vi "probe_pol_mod.vi"() -> ()   [LabVIEW 2011]
uses:
  <vilib>/express/express arith-compare/Formula/XNode/ExpressFormulaBlockNode.xnode
panel:
  out "Right AC":dbl format="%#_5g"
  out "Left AC":dbl format="%#_5g"
  in  "Extract Tone?":bool
  out "Right Amplitude":dbl
  out "Right Freq":dbl
  out "Left Amplitude":dbl
  out "Left Freq":dbl
  out "Pump Status":bool
  in  "Pump Power On?":bool
  out "Right Peak to Peak":dbl
  out "Left Peak to Peak":dbl
  out "Right Ratio":dbl
  out "Left Ratio":dbl
  in  "Shutter":bool
  out "r":dbl
  in  "Number Right Samples":i32=1100
  out "Right Zero Pump On":dbl
  out "Left Zero Pump On":dbl
  out "Waveform Chart":dbl(graph)
  out "Polarization":dbl
  in  "Set Zero":bool
  out "Right Zero":dbl
  out "Left Zero":dbl
  in  "Number Left Samples":i32=2000
  out "Right Mean":dbl format="%#_5g"
  out "Left Mean":dbl format="%#_5g"
  out "Signals":dynamicdata(graph) caption="Section"
  in  "High Signal Start":i32=100 caption="Begin Sample"
  in  "Low Signal Start":i32=1000 caption="Begin Sample"
  in  "stop":bool
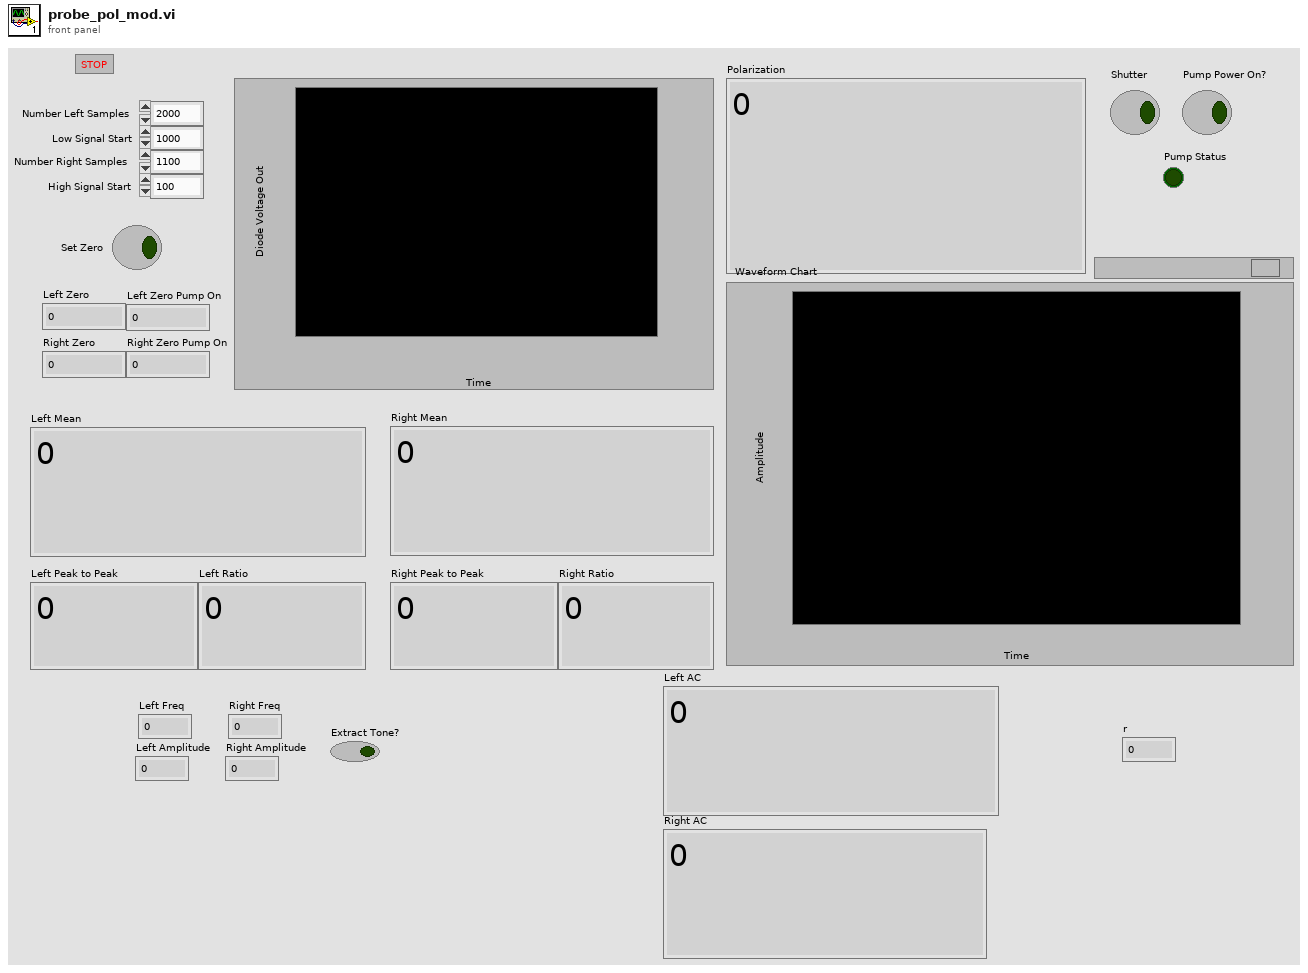
[diagram p1: front panel]
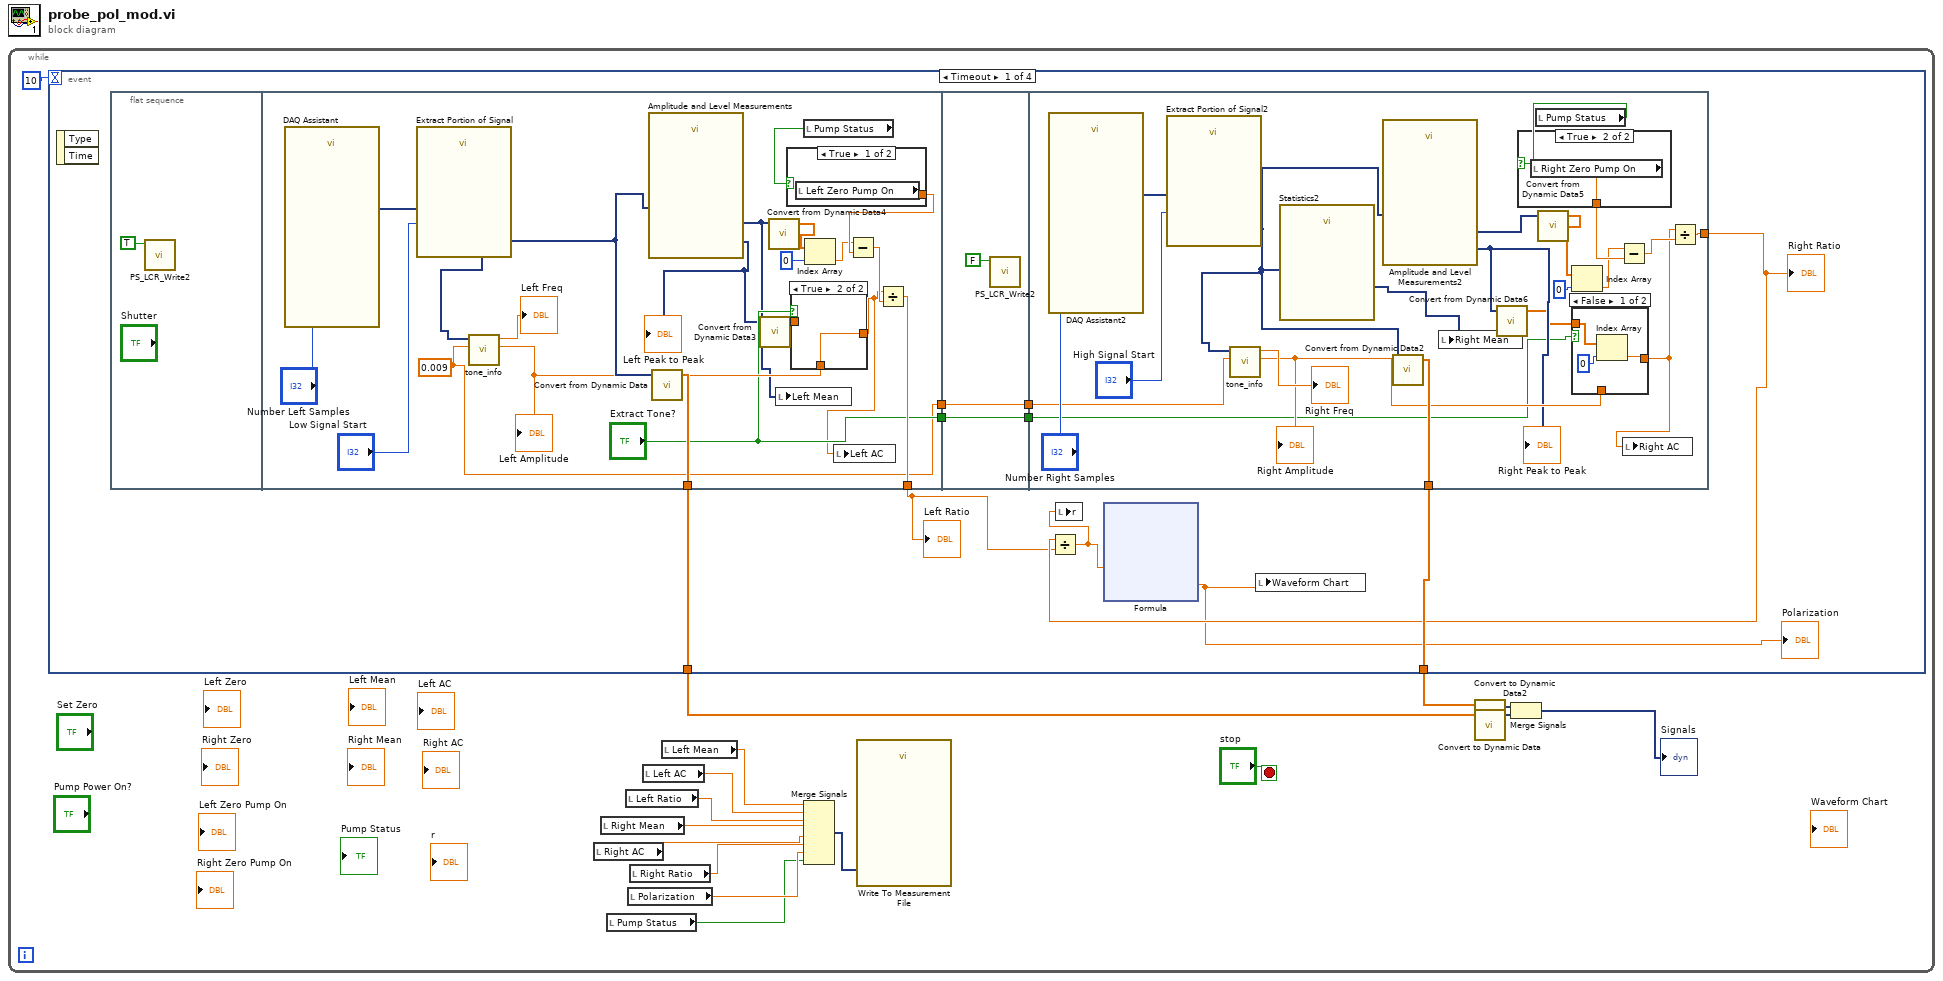
[diagram p0: block diagram]
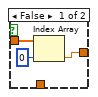
[diagram p2: hidden frame]
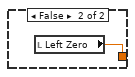
[diagram p3: hidden frame]
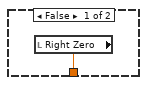
[diagram p5: hidden frame]
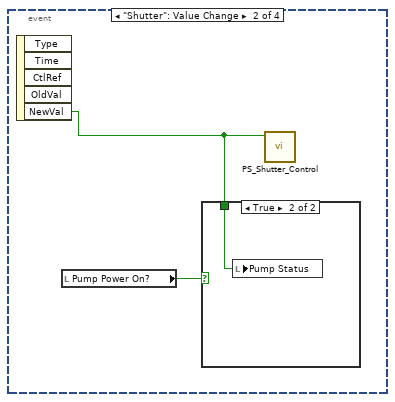
[diagram p6: hidden frame]
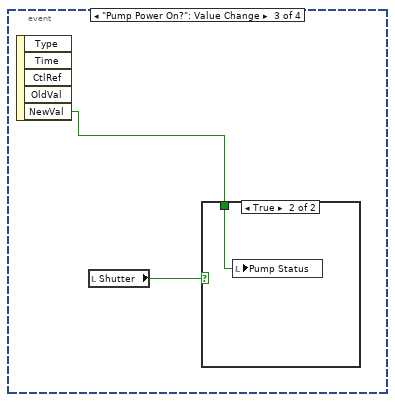
[diagram p8: hidden frame]
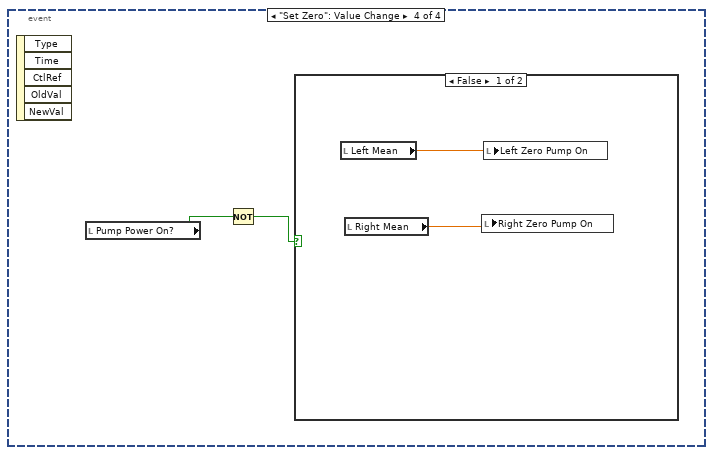
[diagram p10: hidden frame]
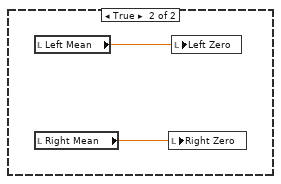
[diagram p11: hidden frame]
diagram:
  n1 = while {
    stop <- "stop" stop-if-true
    n2 = event shown="[0] Timeout" {
      selector: _ -> [_ _ _ _]
      dyn-events: _ -> [_ _ _ _]
      timeout: 10 -> [_ _ _ _]
      tunnel: [w26 _ _ _] -> w14
      tunnel: [w25 _ _ _] -> w12
      event Timeout {
        n3 = event-data() -> ()  [unwired: 1 in, 2 out]
        n4 = flat-sequence {
          tunnel: [w52] -> w26
          tunnel: [w51] -> w21
          tunnel: ["Extract Tone?"] -> w22
          tunnel: [w36] -> w17
          tunnel: [w63] -> w23
          tunnel: w22 -> [w63]
          tunnel: [w62] -> w18
          tunnel: w17 -> [w62]
          tunnel: [w83] -> w25
          tunnel: [w80] -> w24
          tunnel: w23 -> [w67]
          tunnel: w18 -> [w65]
          frame #0 {
            n5 = call "PS_LCR_Write2.vi"("On/Off"=TRUE) -> ()  [unwired: 10 in, 1 out]
          }
          frame #1 {
            w36 = 0.009 ("threshold")
            n6 = call "DAQ Assistant"("number of samples"="Number Left Samples") -> ("data"=w54:dynamicdata)  [unwired: 16 in, 2 out]
            n7 = call "Extract Portion of Signal"("Begin Sample"="Low Signal Start", "Signals"=w54) -> ("Section"=w47:dynamicdata)  [unwired: 8 in, 1 out]
            n8 = call "tone_info.vi"("threshold"=w36, "time signal in"=w47) -> ("amplitude"=w45:dbl, "frequency"=→"Left Freq":dbl)  [unwired: 7 in, 1 out]
            "Left Amplitude" <- w45
            n9 = call "Amplitude and Level Measurements"("Signals"=w47) -> ("Mean (DC)"=w41:dynamicdata, "Peak to Peak"=w42:dynamicdata)  [unwired: 12 in, 1 out]
            "Left Peak to Peak" <- w42
            n10 = call "Convert from Dynamic Data"("Dynamic Data Type"=w47) -> ("Array"=w52:dbl[])  [unwired: 3 in]
            n11 = call "Convert from Dynamic Data3"("Dynamic Data Type"=w42) -> ("Array"=w43:dbl[])  [unwired: 3 in]
            n12 = call "Convert from Dynamic Data4"("Dynamic Data Type"=w41) -> ("Array"=w39:dbl[])  [unwired: 3 in]
            n13 = local write "Left Mean"(w41) -> ()
            n14 = case shown="True" "Extract Tone?" {
              tunnel: [w57 w59] -> w37
              tunnel: w45 -> [_ w59]
              tunnel: w43 -> [w58 _]
              frame False {
                n15 = Index Array(array=w58, index=0) -> (element=w57:dbl)
              }
              frame True {
              }
            }
            n16 = local read "Pump Status"() -> (w50:bool)
            n17 = case shown="True" w50 {
              tunnel: [w60 w61] -> w49
              frame True {
                n18 = local read "Left Zero Pump On"() -> (w60:dbl)
              }
              frame False {
                n19 = local read "Left Zero"() -> (w61:dbl)
              }
            }
            n20 = Index Array(array=w39, index=0) -> (element=w40:dbl)
            n21 = local write "Left AC"(w37) -> ()
            n22 = Subtract(x=w40, y=w49) -> (x-y=w48:dbl)
            n23 = Divide(x=w37, y=w48) -> (x/y=w51:dbl)
          }
          frame #2 {
            n24 = call "PS_LCR_Write2.vi"("On/Off"=FALSE) -> ()  [unwired: 10 in, 1 out]
          }
          frame #3 {
            n25 = call "DAQ Assistant2"("number of samples"="Number Right Samples") -> ("data"=w84:dynamicdata)  [unwired: 16 in, 2 out]
            n26 = call "Extract Portion of Signal2"("Begin Sample"="High Signal Start", "Signals"=w84) -> ("Section"=w75:dynamicdata)  [unwired: 8 in, 1 out]
            n27 = call "tone_info.vi"("threshold"=w65, "time signal in"=w75) -> ("amplitude"=w70:dbl, "frequency"=→"Right Freq":dbl)  [unwired: 7 in, 1 out]
            "Right Amplitude" <- w70
            n28 = call "Statistics2"("Signals"=w75) -> ("Arithmetic Mean"=w82:dynamicdata)  [unwired: 24 in, 2 out]
            n29 = call "Amplitude and Level Measurements2"("Signals"=w75) -> ("Mean (DC)"=w72:dynamicdata, "Peak to Peak"=w69:dynamicdata)  [unwired: 12 in, 1 out]
            "Right Peak to Peak" <- w69
            n30 = call "Convert from Dynamic Data2"("Dynamic Data Type"=w75) -> ("Array"=w83:dbl[])  [unwired: 3 in]
            n31 = local write "Right Mean"(w82) -> ()
            n32 = call "Convert from Dynamic Data6"("Dynamic Data Type"=w69) -> ("Array"=w68:dbl[])  [unwired: 3 in]
            n33 = local read "Pump Status"() -> (w79:bool)
            n34 = case shown="True" w79 {
              tunnel: [w90 w91] -> w77
              frame False {
                n35 = local read "Right Zero"() -> (w90:dbl)
              }
              frame True {
                n36 = local read "Right Zero Pump On"() -> (w91:dbl)
              }
            }
            n37 = call "Convert from Dynamic Data5"("Dynamic Data Type"=w72) -> ("Array"=w74:dbl[])  [unwired: 3 in]
            n38 = Index Array(array=w74, index=0) -> (element=w71:dbl)
            n39 = case shown="False" w67 {
              tunnel: [w87 w89] -> w66
              tunnel: w70 -> [_ w89]
              tunnel: w68 -> [w86 _]
              frame False {
                n40 = Index Array(array=w86, index=0) -> (element=w87:dbl)
              }
              frame True {
              }
            }
            n41 = Subtract(x=w71, y=w77) -> (x-y=w78:dbl)
            n42 = local write "Right AC"(w66) -> ()
            n43 = Divide(x=w66, y=w78) -> (x/y=w80:dbl)
          }
        }
        n44 = Divide(x=w24, y=w21) -> (x/y=w20:dbl)
        n45 = local write "r"(w20) -> ()
        n46 = xnode "Formula"("r"=w20) -> ("Result"=w19:dbl)  [unwired: 1 in, 1 out]
        "Polarization" <- w19
        n47 = local write "Waveform Chart"(w19) -> ()
        "Left Ratio" <- w21
        "Right Ratio" <- w24
      }
      event "Shutter": Value Change {
        n48 = event-data() -> ("NewVal"=w93:bool)  [unwired: 1 in, 4 out]
        n49 = local read "Pump Power On?"() -> (w92:bool)
        n50 = case shown="True" w92 {
          tunnel: w93 -> [_ w94]
          frame False {
          }
          frame True {
            n51 = local write "Pump Status"(w94) -> ()
          }
        }
        n52 = call "PS_Shutter_Control.vi"("On/Off"=w93) -> ()  [unwired: 10 in, 1 out]
      }
      event "Pump Power On?": Value Change {
        n53 = event-data() -> ("NewVal"=w96:bool)  [unwired: 1 in, 4 out]
        n54 = local read "Shutter"() -> (w95:bool)
        n55 = case shown="True" w95 {
          tunnel: w96 -> [_ w97]
          frame False {
          }
          frame True {
            n56 = local write "Pump Status"(w97) -> ()
          }
        }
      }
      event "Set Zero": Value Change {
        n57 = event-data() -> ()  [unwired: 1 in, 5 out]
        n58 = local read "Pump Power On?"() -> (w99:bool)
        n59 = Not(x=w99) -> (.not. x?=w98:bool)
        n60 = case shown="False" w98 {
          frame False {
            n61 = local read "Left Mean"() -> (w101:dbl)
            n62 = local read "Right Mean"() -> (w100:dbl)
            n63 = local write "Right Zero Pump On"(w100) -> ()
            n64 = local write "Left Zero Pump On"(w101) -> ()
          }
          frame True {
            n65 = local read "Left Mean"() -> (w103:dbl)
            n66 = local read "Right Mean"() -> (w102:dbl)
            n67 = local write "Right Zero"(w102) -> ()
            n68 = local write "Left Zero"(w103) -> ()
          }
        }
      }
    }
    n69 = local read "Right AC"() -> (w6:dbl)
    n70 = local read "Right Mean"() -> (w2:dbl)
    n71 = local read "Pump Status"() -> (w1:bool)
    n72 = local read "Left Ratio"() -> (w7:dbl)
    n73 = local read "Polarization"() -> (w4:dbl)
    n74 = local read "Right Ratio"() -> (w5:dbl)
    n75 = local read "Left AC"() -> (w8:dbl)
    n76 = local read "Left Mean"() -> (w3:dbl)
    n77 = Merge Signals(w3, w8, w7, w2, w6, w5, w4, w1) -> (w9:dynamicdata)
    n78 = call "Write To Measurement File"("Signals"=w9) -> ()  [unwired: 16 in, 3 out]
    n79 = call "Convert to Dynamic Data2"("Array"=w12) -> ("Dynamic Data Type"=w11:dynamicdata)  [unwired: 3 in]
    n80 = call "Convert to Dynamic Data"("Array"=w14) -> ("Dynamic Data Type"=w13:dynamicdata)  [unwired: 3 in]
    n81 = Merge Signals(w11, w13) -> (→"Signals":dynamicdata)
  }
